vi "Convert XML Value to VTT.vi"(11 "XML Value":string) -> (3 "VTT Equiv":string)   [LabVIEW 2026, in "VILab.lvlib"]
uses:
  VILab.lvlib
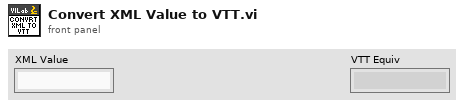
[diagram p1: front panel]
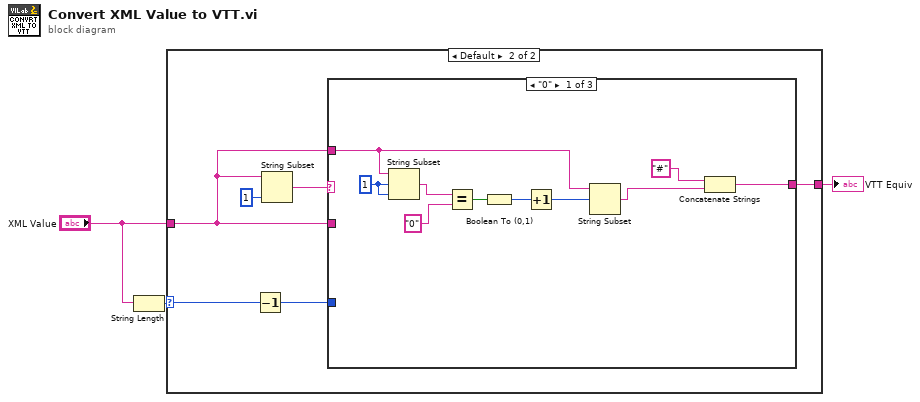
[diagram p0: block diagram]
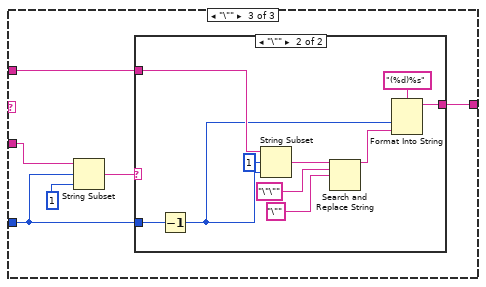
[diagram p4: hidden frame]
diagram:
  n1 = String Length(string="XML Value") -> (length=w3:i32)
  n2 = case shown="Default" w3 {
    selector: w3 -> [_ w9]
    tunnel: [w4 w8] -> w2
    tunnel: "XML Value" -> [w4 w5]
    frame 1 {
    }
    frame Default {
      n3 = Decrement(x=w9) -> (x-1=w6:i32)
      n4 = String Subset(string=w5, length (rest)=1 ("length (rest)")) -> (substring=w7:string)  [unwired: 1 in]
      n5 = case shown="\"0\"" w7 {
        tunnel: w5 -> [w15 w21 w27]
        tunnel: [w13 w21 w26] -> w8
        tunnel: w6 -> [_ _ w23]
        tunnel: w5 -> [_ _ w24]
        frame "0" {
          w20 = 1 ("offset (0)")
          n6 = String Subset(string=w15, offset (0)=w20, length (rest)=w20) -> (substring=w19:string)
          n7 = Equal?(x=w19, y="0") -> (x = y?=w17:bool)
          n8 = Boolean To (0,1)(Boolean=w17) -> (0, 1=w16:i16)
          n9 = Increment(x=w16) -> (x+1=w14:i16)
          n10 = String Subset(string=w15, offset (0)=w14) -> (substring=w12:string)  [unwired: 1 in]
          n11 = Concatenate Strings("#", w12) -> (w13:string)
        }
        frame Default {
        }
        frame "\"" {
          n12 = String Subset(string=w24, offset (0)=w23, length (rest)=1 ("length (rest)")) -> (substring=w22:string)
          n13 = case shown="\"\\\"\"" w22 {
            tunnel: w27 -> [w28 w35]
            tunnel: w23 -> [_ w30]
            tunnel: [w28 w31] -> w26
            frame Default {
            }
            frame "\"" {
              n14 = Decrement(x=w30) -> (x-1=w29:i32)
              n15 = String Subset(string=w35, offset (0)=1, length (rest)=w29) -> (substring=w37:string)
              n16 = Search and Replace String(input string=w37, search string="\"\"", replace string="\"" ("search string")) -> (result string=w34:string)  [unwired: 5 in, 3 out]
              n17 = Format Into String(format string="(%d)%s", w29, w34) -> (resulting string=w31:string)  [unwired: 2 in, 1 out]
            }
          }
        }
      }
    }
  }
  "VTT Equiv" <- w2
